vi "7_1.vi"() -> ()   [LabVIEW 2021, in "2023.lvlib"]
uses:
  2023.lvlib
  CardHand.lvclass
  CardHand.lvclass/CardHand.ctl
  <vilib>/ErrorRing/Error Ring.xnode
panel:
  out "sum":i32
  out "Array 3":refnum<class "CardHand.lvclass">[](array[class])
  out "Indices of Elements":i32[](array[numeric])
  out "Hand_in_array":i32[][](array[numeric])
  out "Numeric":i32
  out "Map":T1(c390)
  out "Hand_Type_Enum":T2(ring)
  out "Array":refnum<class "CardHand.lvclass">[](array[class])
  in  "Demo / Real Input":bool
  # "--- Day 7: Camel Cards ---"
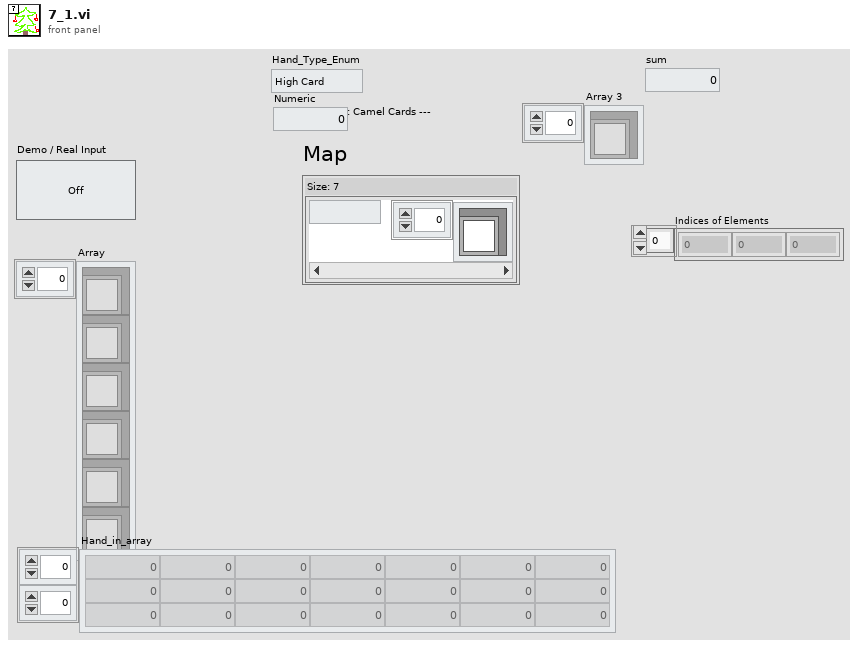
[diagram p1: front panel]
types:
  T1 = map{enum16{"High Card", "One Pair", "Two Pair", "Three of Kind", "Full House", "Four of Kind", "Five of Kind", "ERROR"}, refnum<class "CardHand.lvclass">[]}
  T2 = enum16{"High Card", "One Pair", "Two Pair", "Three of Kind", "Full House", "Four of Kind", "Five of Kind", "ERROR"}
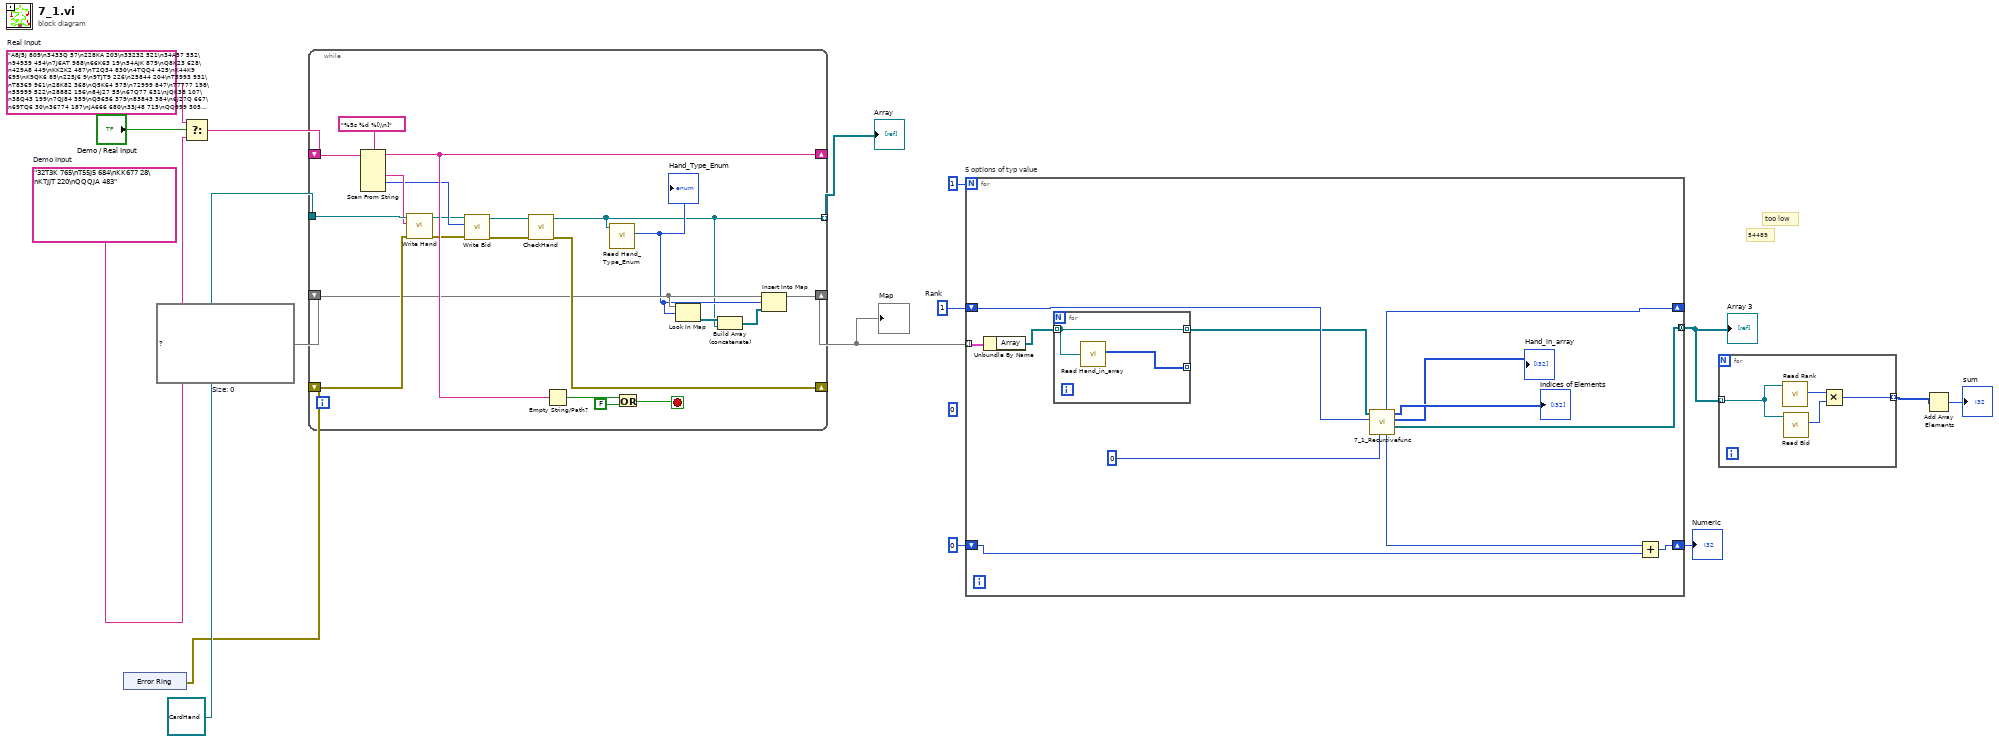
[diagram p0: block diagram]
diagram:
  (unwired) 0
  w7 = 1  # Rank
  w9 = T1 {}  # Size: 0
  w16 = "A8J5J 809\n3433Q 57\n228KA 203\n33232 521\n34A57 552\n94939 454\n7J6AT 988\n66K63 19\n54AJK 879\nQ8K23 628\n429A8 449\nKK2K2 487\nT2Q34 830\n4TQQ4 425\nK44K9 695\nK9QK6 85\n225J6 9\n9TJT9 226\n25844 204\nT3993 931\nT8369 961\n28K82 368\nQ5K64 575\n72999 847\nT7777 198\n55999 522\n28882 156\n84J27 55\n67Q77 631\nJQK38 107\n38Q43 199\n7QJ84 359\nQ5656 379\n83843 384\n6J27Q 667\n69TQ6 30\n36774 187\nJA666 680\n33J48 715\nQQ999 305\n7Q9TJ 870\n453Q7 767\nAKAKK 597\n2JKKT 576\nJKQ2Q 320\nQQTQK 101\nTQ975 468\n6T73K 41\n98A34 11\nJK4AJ 463\n666JJ 742\nT333J 332\n9AK46 880\n324J9 283\n5535Q 224\nQQKKQ 352\n66266 177\nK89K9 458\nTTTT9 649\nKQ935 848\nJ8JJJ 155\n555A6 136\n9QKQ5 309\n6AJ65 964\nA23Q2 862\nK7QA9 241\n43759 265\n66A66 129\nTKKK8 634\n5TKKK 735\nQKKK4 414\n33JTT 95\n63A6A 983\nK78K8 942\n4Q52A 885\nQTAAT 314\nTTTQT 264\n999A9 194\n7JKJA 936\nJ4444 893\nQQAQA 864\nK8888 731\nAAJKK 472\n867T5 729\n9QKJ6 255\n8A5A5 930\nA3KQ3 489\nKK999 664\nQ22QQ 310\nJ8TJ3 105\n4285J 533\nAQQQ2 516\n5755J 793\n2TT2T 12\n78KJ8 873\n995AJ 643\n7977J 990\n295T5 422\nQJ3A4 184\nQQQ26 248\n44848 287\n5J656 315\nQQQ9Q 294\nTQA67 484\n8A662 920\n59393 56\n9997Q 828\nTJ3QJ 277\n2Q277 600\nJKQQT 500\n58888 673\n55522 236\n26887 245\n3JA3A 21\nTK4TK 15\nT38K4 891\nAKQAQ 490\nAJ9QA 452\n44T43 208\nT9Q9J 905\nJQJQ4 574\nAA369 783\nQ8K49 158\n8Q74K 387\n7AAAA 216\nQ5KQQ 68\n54J5K 617\nKK2JK 32\n4A29T 398\n444JJ 517\n9T82Q 531\nT868Q 238\n5585J 52\n9JAK3 456\n26289 295\n3766J 622\nKKTAK 147\n9J46K 334\n739QT 512\n8TTQ5 252\n78957 162\n555J5 13\nA3858 14\nJ9JJ9 662\nKK8KK 424\nQTQTT 871\n5TT5J 20\n8897A 342\n99J9T 884\nT6J78 710\nATTTA 934\nTTJ63 346\nA4325 290\n5K7K7 83\nQQA96 605\n8K8KK 693\n82885 232\n8A3A2 38\nKJQ93 802\n34TTT 829\n6T2TQ 406\n748J4 826\nAJ555 530\nQ4K48 994\n48948 223\n74666 181\n49444 278\n54886 470\n99A7A 803\n4784Q 543\n4AK3T 747\nT9J8Q 306\nQ4K77 275\nQ3QQQ 672\nA237J 459\n3J333 776\nJJJK5 349\n5Q455 619\n343AA 71\n97777 817\n69669 835\n85J45 766\nTT2TA 998\n5555Q 34\nKT245 620\n5T7AA 93\nKKK36 432\n5QQJ4 956\nA375A 79\nQ9229 948\nJQ33Q 291\n858A8 925\nT4JKT 892\n366Q9 240\n2J8QQ 967\n66646 243\n68866 726\nTTJAT 682\n3A248 446\n33373 122\n6J866 813\nQ9QK9 404\n2TTT9 49\nA28K7 935\nKA458 467\n333A3 451\n7A7AJ 402\n6K9T9 852\n77747 426\nJQK53 661\n4T455 653\nQ5527 109\nK3399 822\n78A9T 161\n454J5 423\n49T86 630\n77778 537\n722JJ 955\nQ248J 760\n3J26A 725\n3533J 593\nT7T7Q 568\nJ7JQQ 298\n3K878 66\n94994 272\n44344 175\n66Q64 688\n7J737 811\n2J84A 113\nJT9T4 51\nKKJ7K 103\n5T5TT 50\n8858Q 455\n276Q7 410\n257K3 656\nK33K3 330\nT6TQ6 97\n999K9 82\n63K29 491\n365A6 508\n2JJKK 609\nAA6K9 765\n7K968 808\n25J7T 46\n6J6K5 538\n9J997 173\nQKKQT 583\n32KJQ 897\nK4935 933\n28228 125\n7Q3J2 326\nKTT36 148\n38344 999\n77757 502\n86JQT 556\n8578J 706\nJJ333 134\n4QQQQ 746\n8QK3K 774\nQ56K9 995\nKT3JK 604\nQJKJ2 348\n6767T 81\nJKKKQ 572\n222K8 607\n55222 972\n6769A 889\n79379 89\nKAJKK 73\nKJJ43 997\n79768 569\nJ7A4A 946\nQ6Q39 911\nJ2Q49 202\n77229 96\n3T333 63\n49T25 912\nAA96A 676\nTT6JT 201\n999Q9 954\nT7A64 899\nJK6KK 338\n6Q77K 60\nJ7TTT 260\nK2QQQ 791\n26766 703\n24QQA 843\n34333 638\n99696 769\nQ7977 952\n733JA 883\nT7AAA 128\nQQQQT 624\n523QT 347\nQ8888 337\n23Q25 602\n548KT 886\n2K9A5 100\nQAQQQ 420\n28494 486\n96A9K 868\nA66AA 623\nQ9Q9Q 658\n6QJ6K 412\nA7A6T 311\nTT8J8 984\n954A3 59\n37A8K 273\nJ3QJQ 753\n97999 78\nT2279 118\n37377 281\n555J4 687\nA46K6 657\n8KAK8 429\n63643 344\n96857 797\n76644 394\nQQAAA 135\n7265T 58\nT67T3 421\n689J6 681\nJ3424 720\n8KJJA 356\n5J599 416\nQ37J9 377\n4J9QQ 409\n45555 939\nA727J 646\nA65JT 981\nTT9JJ 618\n626T5 647\n74TA7 211\n6389K 824\n9QA9A 759\nJ36JJ 932\nAQA7A 877\n9AAJ9 444\nAQ7AQ 4\n4JJ6J 428\n6K3K6 689\n875KJ 866\nT77TT 323\n8QJ32 612\nQQKQQ 700\nQ9444 782\n68K9J 979\nA4AAK 367\n8JA8K 288\n69QJA 540\nJQJ85 80\n82Q39 498\n74772 962\n99922 76\nKAK84 197\n66866 152\n54445 189\n57J7J 328\n3ATTT 745\n6K646 92\nT63A5 785\n3T9KA 974\nQ85QQ 770\n3KK2K 527\n8772J 473\nJAJ55 854\n7529K 844\n33493 819\n279J8 106\n4KK8J 563\n5K5K5 751\n7QK62 945\n794A7 704\n46QT2 548\nJ77T7 364\nA5A5J 639\nT66TJ 382\nAA8KT 784\nK5K4A 296\nJ55J5 598\nQ7Q77 985\n78774 965\n398T7 141\n9848T 771\n47584 124\n7JT47 924\nT6999 392\n977JQ 709\nT4K62 860\n7K722 362\nA7JAA 787\n4T4JJ 549\n5J92J 616\nQJT27 901\n58558 53\n555K5 851\n57457 84\nJJ842 450\nA3KAK 381\nAAQJJ 67\n985T9 378\nQ899J 737\nKA549 363\n75K2J 102\n9K9Q9 497\n33533 991\n9QK6T 743\n94652 115\n642T3 27\n4J299 730\n5KK3K 535\n9J588 748\n63472 867\n98K6A 215\nK9J4K 744\n58255 825\n99969 831\n22Q68 324\nA6665 926\nKJJAT 679\n392J7 739\nJ65T6 775\n2AA8A 881\n69666 166\nQ969J 896\n22893 698\nJKK33 509\n4JJ46 779\n33222 374\nAJA22 515\n7669J 603\n73787 504\n33858 959\n34T2J 857\nTKQQ9 485\nA9T34 723\n4KQQQ 389\nJQ2Q5 112\n93T33 529\nQQ5QQ 233\n42949 507\n5K553 466\n44KKJ 1000\n6J783 42\n822A8 592\n48847 116\nAJA7T 505\n44J24 214\n55454 274\n2KA84 914\n4TT24 788\n3J553 221\nA5687 307\n73388 169\n67667 798\n992JQ 335\nQ6665 846\nK9KAK 354\nTAQ72 518\n72727 210\n99929 875\n7J777 75\n22J22 650\n6AJ5A 258\n85J4J 834\nKT2J3 462\nJ59KT 461\nQQTTQ 841\nJ4488 413\nJJ5K5 941\n5KQT3 733\n64Q4K 254\n4JJ77 327\nJA22K 270\n47444 850\n73956 577\nKKK33 977\nKKK3K 978\nAAAAJ 614\nQ3KQ3 371\n23J22 878\nKQ5A3 532\nK3KKA 235\n2Q48Q 481\n25A58 626\nAK7AA 810\nQ8T8Q 457\n2TT83 206\n8Q985 176\nJA54Q 436\n88J88 859\nTKTTK 890\n787AA 902\n3882J 393\nJAT77 244\n994J7 207\nQ8898 579\nJ8A8A 973\n595KT 121\n7232K 718\nQA3QJ 212\n9A92A 351\nATAJ4 669\nQ3QA3 494\n54779 159\n37J33 495\n6QQQK 943\n9KKKK 832\nT99TT 714\nK4AJ3 659\n29959 580\nKK55Q 37\n8JJ44 345\nA987J 686\n4T5JJ 544\n44KA4 247\n946Q2 234\nQ299Q 976\nQQ497 70\n6578K 31\n8J85J 469\nTT8A2 690\nJJA99 573\nK3TTT 590\n2JTQK 479\n858Q4 738\n242J2 45\nA942K 292\n4A242 431\n599K4 699\n7J579 665\n55599 482\n75Q5J 26\n99994 523\n6QQJQ 33\n65556 895\n898TA 794\nJ4AA9 853\n392J9 578\n7Q333 228\n4JKTJ 558\n4443J 929\nKA5A6 944\nK29J4 433\n88788 17\nJJ737 493\n27T27 692\n97877 526\nK4848 888\nQ954A 958\nA4A44 25\nQAAAJ 419\nKKJ4T 546\n59946 140\n8T2JK 395\n237AK 253\n84Q44 553\n78788 353\nJ925T 585\nJAJAA 227\nJTAAT 539\n99777 139\nTT938 213\nJ6665 163\n77A55 62\n7QA5J 179\nT3K33 361\n4KJ46 773\n55A88 637\n7TJ28 684\nA77A7 719\n585AT 443\n4J92J 2\nJQQ77 110\nJ2KKA 629\nAA5A8 313\n6AJAA 496\nK9KJ9 987\nQQTT8 968\n8J82T 732\n347J3 144\n22277 560\nTJKKT 302\n5Q522 229\n7K778 127\n66J66 126\n98J92 608\nJKK28 863\n96955 249\n2K5Q8 752\nK52A3 601\n93Q86 506\n93264 754\n333T8 411\n92J92 172\n22722 615\n48TQ2 476\n49524 645\n844T3 276\n99JKA 408\n92293 74\n87T92 816\nQ9A75 72\nT3TTT 18\n98888 635\n838J3 117\n222AA 741\n44446 90\nTT2J2 150\n65222 777\n999JJ 534\n2A2T6 937\nJJJJJ 10\n27A27 230\n24444 606\n87778 778\nTA8QJ 839\n5TTTT 336\nK78JT 519\nA5KA5 865\n42255 503\n99J99 908\n373J8 492\n63863 947\n5JK32 390\n33399 711\n6444K 722\n99J94 143\n82Q2Q 792\n6JQ64 555\n9Q85K 188\nK378T 960\n39268 119\nAJA2Q 1\n32333 547\n5A55Q 584\n89896 904\n22226 318\nQ292Q 511\nKKKKJ 86\n2KJK2 677\n86K35 663\nA8Q9J 403\nQ6T6Q 499\nA4JJ4 807\n8QT57 405\n7A744 385\n5K5KK 399\n64966 827\nJ992J 133\n24466 154\nAAQJQ 316\nTT8TK 586\n9K7AK 587\n667JJ 910\nJQQQQ 400\n8444J 528\n4QQ4A 858\nKK598 246\nAATAT 445\nJ756A 837\nTJ632 916\nT4697 913\n2J225 474\n6JKKJ 146\n57498 372\n2222A 7\nQ444A 750\nA4AAJ 660\nTQ548 876\nJJQQQ 697\n7A777 375\nQQQQ7 98\n65656 65\n57757 763\nA53K6 957\n2K8KK 191\n666K7 370\nJ77TT 872\nJTT75 786\n57494 749\n648A6 887\n3982A 48\n9A2JJ 820\nKJ5T5 724\nA773A 918\nK6754 488\n8A58A 442\n88AA8 845\nK3K5J 909\n8JJ8T 123\n555AA 756\nK33J3 514\n57975 861\n386K2 167\nJ9783 927\n27744 383\n2J6Q8 707\n2KQT8 823\n766J6 196\n4A499 717\n6J524 708\n744K7 683\n2Q22A 396\n3Q9T8 138\n884TJ 192\nK6898 321\n6K446 29\n85634 427\n5J588 559\n96J96 678\nKQQ3T 833\nAJ755 369\n444T4 550\n68277 267\nAJ7J4 373\nQ4Q4Q 652\n22822 582\n36K79 195\n9797T 286\n89999 460\n66J33 636\n55888 640\n53693 716\n39KJ8 762\n55K59 796\n96JKK 183\n55855 268\nJ4K83 285\nKK7KK 299\nKKKKT 940\nJ77J7 906\n88TTT 388\n5T54J 111\nT8QA9 806\n22K22 256\nJT228 970\n79624 322\nKKK77 69\n88JJ8 91\nA222T 132\n67JA7 312\n77767 971\n869J2 471\n9T998 595\nJA266 64\n2272T 755\n9K7J6 22\n254T5 849\n82T9J 289\nQ76TJ 331\nTQQT6 5\n77737 536\n7T783 567\n8T888 705\n6T53K 186\nQ6K57 301\n78Q78 130\n5K656 293\n33J32 339\n66J96 894\n57J53 581\n6K554 217\nKKJKJ 696\n5AAA5 789\n29429 44\n5K552 969\n8442T 928\n84444 137\nT9J48 557\n56KA8 386\n7QQ27 764\nA828A 165\nAA699 641\n79922 570\nJA5T8 407\n449QJ 651\n5555T 43\n5TK97 907\n78487 478\nQQQ55 448\n88848 938\n3J55T 99\n6J94A 16\n99K97 358\n34643 818\n226K6 88\n62226 415\nT3633 758\nK2KA9 350\n4K968 903\n9TKA4 284\n7T274 220\nTTJTT 108\n8J625 589\nJQKQQ 28\n5AJ59 209\nJ779K 239\nQQQ2Q 795\n836KT 477\nA4432 8\n8998J 855\n7JJJA 882\n44646 303\nJ9A2A 781\nQKKQ2 721\nQ8Q2Q 898\n6464Q 297\nT99QA 993\n82K9A 953\n36667 453\n383QQ 120\n37J49 193\n7T758 805\nJ5TTT 170\n8AAJQ 36\nAT7TJ 632\nT777A 6\n833A9 917\nA254K 992\nA4QTQ 259\n88522 480\n7J3JJ 836\n5453T 366\n7J2JT 613\nAATT4 47\nK99J3 757\n567Q8 114\nA9AAA 242\nJJ343 218\n3Q66Q 87\n35A62 231\n2J924 250\n4TTQ4 430\n2QKJ8 279\nQ7555 257\nTTT7T 520\n4TT45 922\nT2375 610\n2J5QA 465\n99498 145\nTTKTQ 205\n26358 674\n66622 727\n66446 821\n6K686 975\n653Q2 963\nJ2A26 772\n88288 761\n5T57T 986\n2QA9A 269\nJTT79 666\nA2KKK 571\n346JK 261\n9K9A9 3\nT3A6T 341\n22422 701\nT7KJA 838\nK4KA3 541\nA94TJ 435\n7JQ59 982\n54444 633\n4J5Q6 280\n7TAA2 365\nJ52J6 447\nTT777 513\nJ8789 740\n256JT 524\nAK44K 317\nK6T6K 171\n9JJ22 648\n33JAK 525\nT988T 262\n2JQQ2 685\n5T8TJ 736\n6K2J8 542\n75AT8 554\n59J5J 185\n88886 153\nJ2727 734\n3K95T 562\n7J677 376\nJT4QJ 856\n923Q7 190\nT43TJ 713\nA975T 160\n4KT95 921\n63QT2 804\nATTTT 77\n39Q99 142\nAKAAK 801\n99444 790\n59953 915\n78522 545\n63J6J 54\n4553Q 40\nA3KJ8 510\nJ4449 627\nJ8J48 815\n68383 923\n98889 325\nJK9KQ 61\n3653J 434\nQ8QQQ 401\nAAAAK 174\n35J55 642\n4T5JK 588\nJ7QK7 439\n55A9A 966\nK2K26 800\nAKT32 304\nQ6Q6J 599\n37JJ3 418\n5227J 23\nJJ62A 440\n2K888 437\nQTQ7J 380\n3J25J 104\n46342 157\n336K7 180\n4444A 168\nAQ686 391\nTQTJQ 591\nJ4456 441\n5T5T5 949\n693A4 266\n92JTJ 654\nT4QA8 768\nATAAA 814\nKK46Q 329\n36366 951\n88348 670\nAATQQ 24\nTTQ8T 980\n56TTT 625\n99J86 668\n55552 438\n25934 675\nAJQQQ 996\nJ2323 263\n9QQQA 712\n4Q7K4 360\nQ958T 308\n55542 35\n68459 164\nK5427 475\n858KK 357\n85Q75 251\n85587 596\n99K22 483\nA4555 182\nQ2337 919\n96784 900\n7J53Q 333\n6J82A 869\n4QQJ4 151\n586K5 464\nKT36J 551\nKKK84 566\n92AQ8 149\nK369Q 340\n2QQTQ 178\nJ3T35 564\nK2TQ9 644\nT7TKA 655\nQ4Q44 840\nQ83TA 282\n6456T 417\nA6AAA 39\nQ74JA 237\n2222T 702\n5A444 271\n82448 222\n6TJ55 694\n56699 131\nAT936 671\n522JT 842\n45T55 200\n8AQ44 691\n6TAAT 728\nJQ245 501\n389T3 225\n33933 300\nA696A 561\n37367 343\n9KJKK 812\n388A8 611\n3TTJT 565\nT5KKT 874\nT3J9J 950\n33Q33 780\nQ2876 799\nK76T6 319\n3QT23 594\n7AA7A 621\nT7757 355\nTT44T 94\nKKK2K 397\nKKKK6 989\nAAA42 219"  # Real Input
  w15 = "32T3K 765\nT55J5 684\nKK677 28\nKTJJT 220\nQQQJA 483"  # Demo Input
  # "too low"
  # "54489"
  n1 = xnode "Error Ring"() -> ("error out"=w11:errorcluster)
  n2 = Select(t=w16, s="Demo / Real Input", f=w15) -> (s? t:f=w13:string)
  n3 = while {
    shift-right: [w34] -> _
    shift-left: w13 -> [w37]
    tunnel: refnum<class "CardHand.lvclass"> refnum ("2023.lvlib:CardHand.lvclass") -> [w33]
    shift-right: [w23] -> _
    shift-left: w11 -> [w31]
    tunnel: [w18] -> w10 mode=indexing
    shift-right: [w17] -> w8
    shift-left: w9 -> [w22]
    stop <- w26 stop-if-true
    n4 = Scan From String(format string="%5s %d %[\\n]", input string=w37) -> (remaining string=w34:string, output 1=w32:string, output 2=w30:i32)  [unwired: 6 in, 2 out]
    n5 = call "Write Hand.vi"("error in (no error)"=w31, "Hand"=w32, "CardHand in"=w33) -> ("error out"=w28:errorcluster, "CardHand out"=w29:refnum<class "CardHand.lvclass">)  [unwired: 7 in]
    n6 = call "Write Bid.vi"("error in (no error)"=w28, "Bid"=w30, "CardHand in"=w29) -> ("error out"=w24:errorcluster, "CardHand out"=w27:refnum<class "CardHand.lvclass">)  [unwired: 7 in]
    n7 = call "CheckHand.vi"("error in (no error)"=w24, "CardHand in"=w27) -> ("error out"=w23:errorcluster, "CardHand out"=w18:refnum<class "CardHand.lvclass">)  [unwired: 8 in]
    n8 = Empty String/Path?(string/path=w34) -> (empty?=w35:bool)
    n9 = call "Read Hand_Type_Enum.vi"("CardHand in"=w18) -> ("Hand_Type_Enum"=w21:T2)  [unwired: 8 in, 2 out]
    "Hand_Type_Enum" <- w21
    n10 = Or(x=w35, y=FALSE) -> (x .or. y?=w26:bool)
    n11 = Look In Map(map=w22, key=w21) -> (value=w20:refnum<class "CardHand.lvclass">[])  [unwired: 1 in, 1 out]
    n12 = Build Array (concatenate)(w20, w18) -> (w19:refnum<class "CardHand.lvclass">[])
    n13 = Insert Into Map(map in=w22, key=w21, value=w19) -> (map out=w17:T1)  [unwired: 2 out]
  }
  "Array" <- w10
  "Map" <- w8
  n14 = for "5 options of typ value" {
    N: 1 -> [_]
    tunnel: w8 -> [w49] mode=indexing
    shift-right: [w38] -> _
    shift-left: w7 -> [w48]
    shift-right: [w45] -> w5
    shift-left: 0 -> [w44]
    tunnel: [w43] -> w4 mode=concatenating
    n15 = Unbundle By Name(w49) -> ("Array"=w47:refnum<class "CardHand.lvclass">[])
    n16 = for {
      tunnel: w47 -> [w50] mode=indexing
      tunnel: [w50] -> w42 mode=indexing
      tunnel: [w51] -> _ mode=indexing
      n17 = call "Read Hand_in_array.vi"("CardHand in"=w50) -> ("Hand_in_array"=w51:i32[])  [unwired: 8 in, 2 out]
    }
    n18 = call "7_1_Recursivefunc.vi"("disabled index (col)"=0, "Rank"=w48, "Array in"=w42) -> ("Array out"=w43:refnum<class "CardHand.lvclass">[], "Hand_in_array out"=→"Hand_in_array":i32[][], "Indices of Elements"=→"Indices of Elements":i32[], "Numeric"=w46:i32, "Rank 2"=w38:i32)  [unwired: 4 in]
    n19 = Add(x=w46, y=w44) -> (x+y=w45:i32)
  }
  "Numeric" <- w5
  "Array 3" <- w4
  n20 = for {
    tunnel: w4 -> [w55] mode=indexing
    tunnel: [w52] -> w3 mode=indexing
    n21 = call "Read Rank.vi"("CardHand in"=w55) -> ("Rank"=w54:i32)  [unwired: 8 in, 2 out]
    n22 = call "Read Bid.vi"("CardHand in"=w55) -> ("Bid"=w53:i32)  [unwired: 8 in, 2 out]
    n23 = Multiply(x=w54, y=w53) -> (x*y=w52:i32)
  }
  n24 = Add Array Elements(numeric array=w3) -> (sum=→"sum":i32)
